vi "Read FindMeasurementsInAppData.vi"(8 "error in (no error)":errorcluster, 11 "Controller Configuration in":refnum<class "Controller Configuration.lvclass">) -> (0 "error out":errorcluster, 2 "FindMeasurementsInAppData":bool, 3 "Controller Configuration out":refnum<class "Controller Configuration.lvclass">)   [LabVIEW 2016, in "Fcn Configuration.lvlib" / "Controller Configuration.lvclass"]
uses:
  <userlib>/Common Components/FCN Configuration/Controller Configuration.lvclass
  <userlib>/Common Components/FCN Configuration/Controller Configuration.lvclass/Controller Configuration.ctl
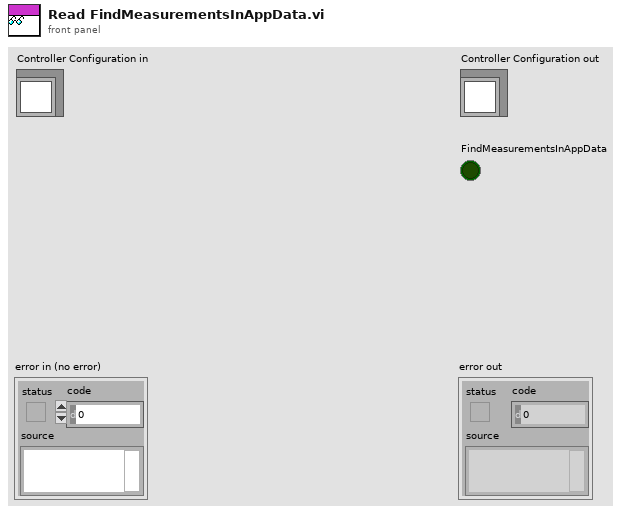
[diagram p1: front panel]
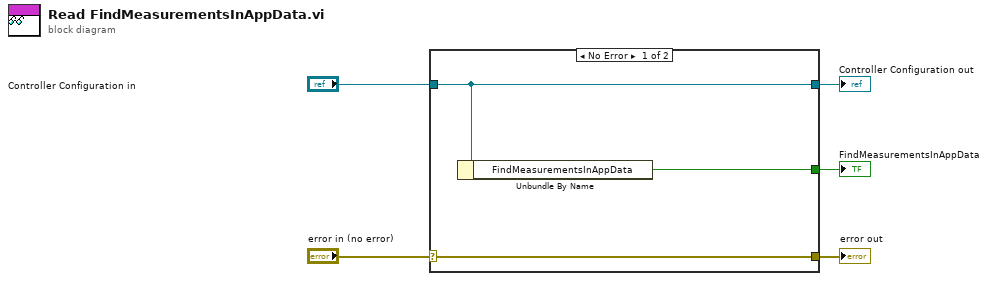
[diagram p0: block diagram]
diagram:
  n1 = case shown="No Error" "error in (no error)" {
    selector: "error in (no error)" -> [w8 w9]
    tunnel: [w8 w9] -> w4
    tunnel: [w7 w10] -> w2
    tunnel: "Controller Configuration in" -> [w7 w10]
    tunnel: [w6 _] -> w1
    frame No Error {
      n2 = Unbundle By Name(w7) -> ("FindMeasurementsInAppData"=w6:bool)
    }
    frame Error {
    }
  }
  "error out" <- w4
  "Controller Configuration out" <- w2
  "FindMeasurementsInAppData" <- w1
